vi "KeithMeterTest.vi"() -> ()   [LabVIEW 2017]
uses:
  <vilib>/Instr/_visa.llb/GPIB Status Boolean Array.ctl
panel:
  out "ibsta 2":T1
  out "ibsta":T1
  in  "address list":i16[](array[numeric])
  out "error out":errorcluster
  out "data string 2":string
  in  "data string":string
  in  "mode":i16
  in  "address":i16=16
  in  "bus":i32
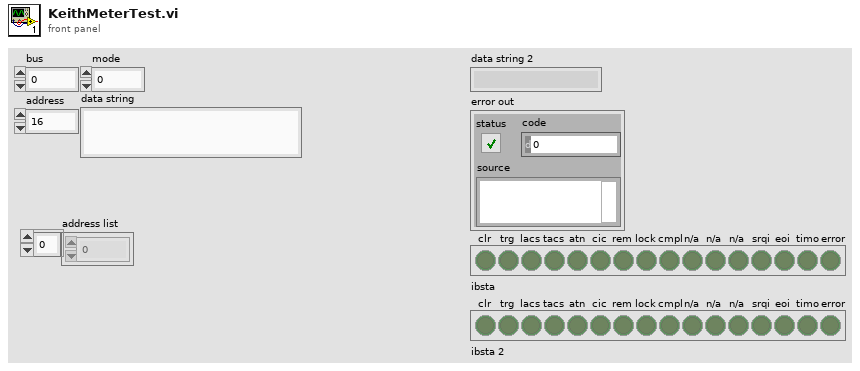
[diagram p1: front panel]
types:
  T1 = typedef "GPIB Status Boolean Array.ctl" = bool[]
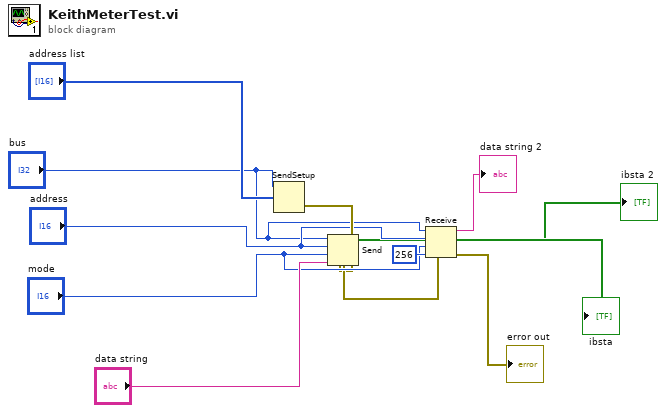
[diagram p0: block diagram]
diagram:
  n1 = SendSetup(3:"address list", 4:"bus") -> (0:w6:errorcluster)  [unwired: 1 in, 1 out]
  n2 = Send(0:"bus", 2:"address", 3:"mode", 4:w6, 5:"data string") -> (6:→"ibsta":bool[], 8:w8:errorcluster)  [unwired: 1 out]
  n3 = Receive(4:w8, 6:256 ("count"), 7:"mode", 8:"address", 9:"bus") -> (0:→"error out":errorcluster, 2:→"ibsta 2":bool[], 3:→"data string 2":string)  [unwired: 1 out]
